vi "PPMS_ScanCampo.vi"(6 "error in (no error)":errorcluster, 7 "Index":i8) -> (0 "error out":errorcluster, 1 "resulting string 2":string="End scan field", 2 "resulting string 1":string="Scan Field from 0.000Tesla to 0.500Tesla at 1.000Tesla/min, in 50 steps, Driven", 3 "Cancelled?":bool)   [LabVIEW 2017]
doc: "Use this template to create a dialog box. This template polls the state of the buttons on the front panel and does not use events. Use the Dialog Using Events template (not available in Base package) to create a dialog box with event handling."
panel:
  in  "Modo de barrido":i32(ring) items=["Solo ir", "Ir y volver"]
  out "Field Mode":i32(ring)=1 items=["Persistent", "Driven"]
  in  "Approach":i32(ring)=1 items=["Linear", "NoOvershoot", "Oscillate"]
  in  "Rate (T/min)":dbl=1.0
  in  "# puntos":u32=50 min=1
  in  "Campo Final (T)":dbl=0.5
  in  "Campo Inicial (T)":dbl
  in  "Cancel":bool
  in  "OK":bool
  # "Noviembre 2020 V1.3  a-sslcdms"
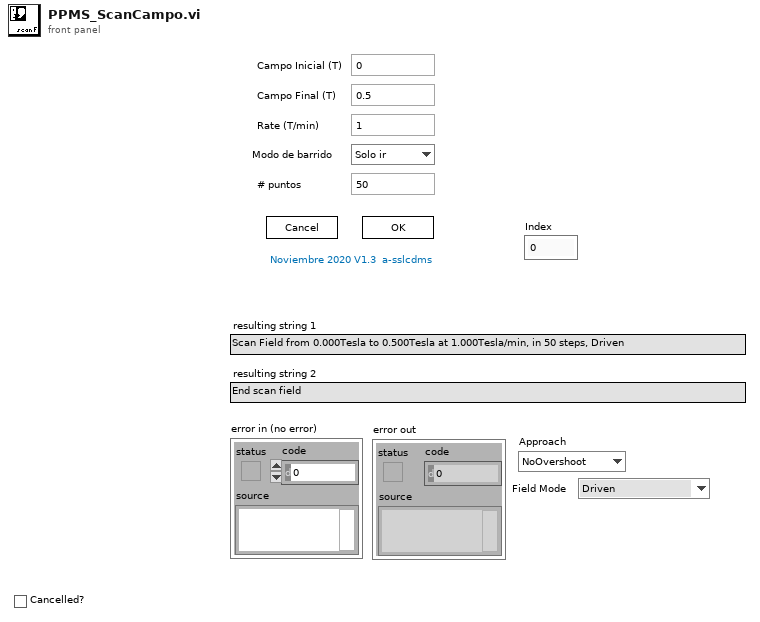
[diagram p1: front panel]
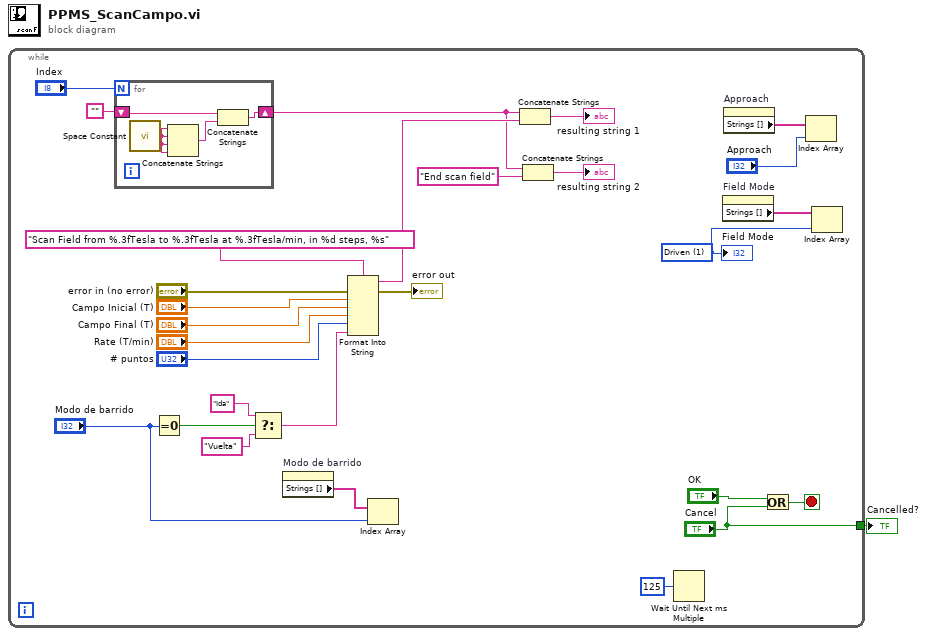
[diagram p0: block diagram]
diagram:
  n1 = while {
    tunnel: ["Cancel"] -> w1
    stop <- w28 stop-if-true
    w8 = 1 items=["Persistent", "Driven"] ("Field Mode")
    n2 = for {
      N: "Index" -> [_]
      shift-right: [w32] -> w16
      shift-left: "" -> [w31]
      n3 = call <vilib>:"Space Constant.vi"() -> ("String"=w30:string)
      n4 = Concatenate Strings(w30, w30, w30, w30) -> (w33:string)
      n5 = Concatenate Strings(w31, w33) -> (w32:string)
    }
    n6 = Equal To 0?(x="Modo de barrido") -> (x = 0?=w7:bool)
    n7 = Select(t="Ida" ("resulting string 2"), s=w7, f="Vuelta" ("resulting string 2")) -> (s? t:f=w4:string)
    n8 = property on="Modo de barrido" class="Ring (strict)"() -> ("Strings []"=w2:string[])  [unwired: 2 in, 2 out]
    n9 = Format Into String(format string="Scan Field from %.3fTesla to %.3fTesla at %.3fTesla/min, in %d steps, %s", error in="error in (no error)", "Campo Inicial (T)", "Campo Final (T)", "Rate (T/min)", "# puntos", w4) -> (resulting string=w20:string, error out=→"error out":errorcluster)  [unwired: 1 in]
    n10 = Index Array(array=w2, index="Modo de barrido") -> ()  [unwired: 1 out]
    n11 = Concatenate Strings(w16, w20) -> (→"resulting string 1":string)
    n12 = Concatenate Strings(w16, "End scan field" ("resulting string 2")) -> (→"resulting string 2":string)
    n13 = Wait Until Next ms Multiple(millisecond multiple=u32 125) -> ()  [unwired: 1 out]
    n14 = property on="Field Mode" class="Ring (strict)"() -> ("Strings []"=w9:string[])  [unwired: 2 in, 2 out]
    n15 = property on="Approach" class="Ring (strict)"() -> ("Strings []"=w14:string[])  [unwired: 2 in, 2 out]
    n16 = Or(x="OK", y="Cancel") -> (x .or. y?=w28:bool)
    n17 = Index Array(array=w14, index="Approach") -> ()  [unwired: 1 out]
    n18 = Index Array(array=w9, index=w8) -> ()  [unwired: 1 out]
    "Field Mode" <- w8
  }
  "Cancelled?" <- w1
